vi "QDM matlab saver_morefreqs_rt_2.vi"(6 "img data stack Input":dbl[][](array[numeric]), 7 "matlab path":path, 8 "Height":i64(slide)=1200 min=0 max=1200 step=4 scale=0.0..1200.0, 9 "Width":i64(slide)=1920 min=0 max=1920 step=4 scale=0.0..1920.0, 10 "freq list (Hz)":dbl[](array[numeric]), 11 "sweep #":i32) -> ()   [LabVIEW 2018]
panel:
  in  "numFreqs":i32=51
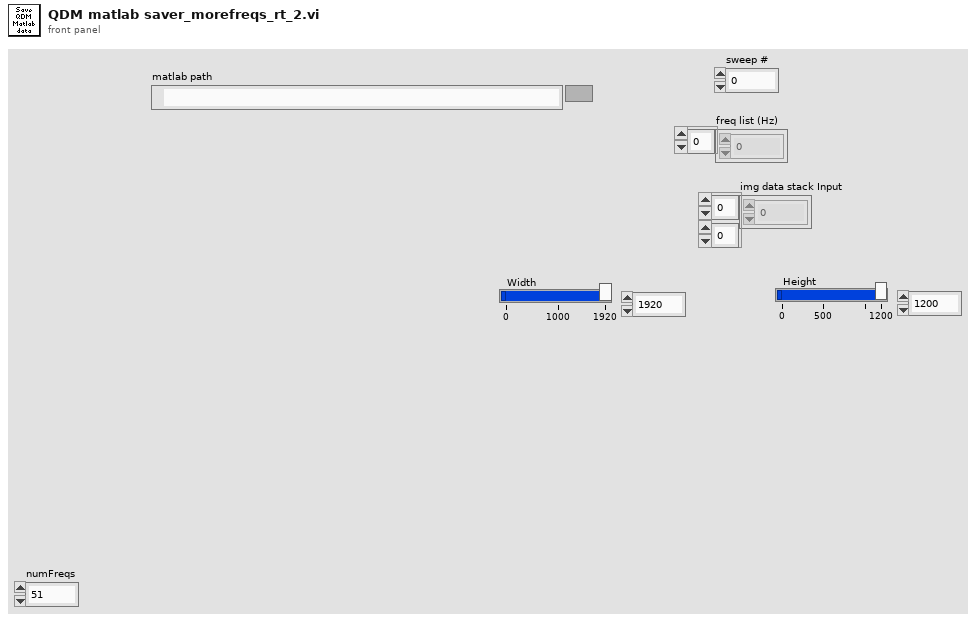
[diagram p1: front panel]
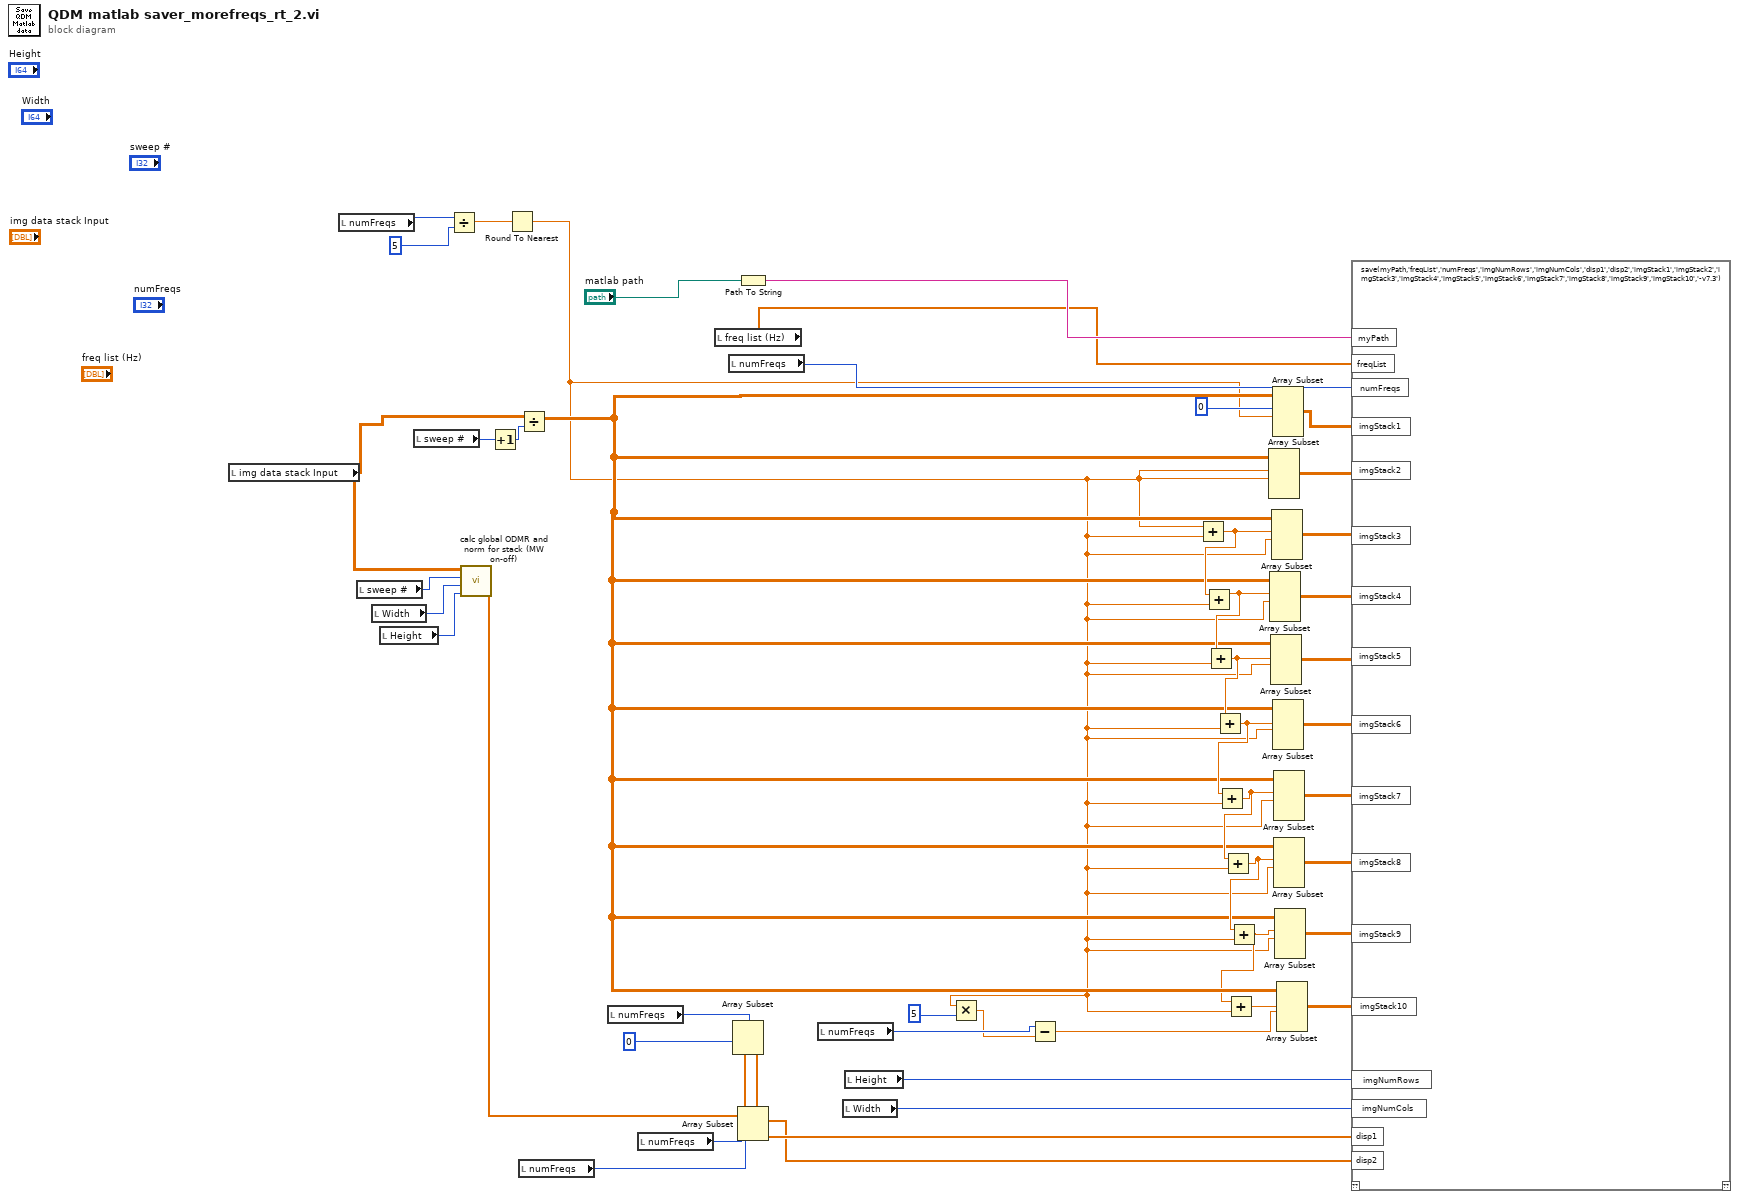
[diagram p0: block diagram]
diagram:
  n1 = local read "img data stack Input"() -> (w37:dbl[][])
  n2 = local read "numFreqs"() -> (w27:i32)
  n3 = local read "sweep #"() -> (w38:i32)
  n4 = local read "Width"() -> (w42:i64)
  n5 = local read "Height"() -> (w43:i64)
  n6 = local read "sweep #"() -> (w40:i32)
  n7 = Divide(x=w27, y=5) -> (x/y=w26:dbl)
  n8 = call "calc global ODMR and norm for stack (MW on-off).vi"("Height"=w43, "Width"=w42, "sweep #"=w38, "img data stack"=w37) -> ("normed spectrum"=w41:dbl[])  [unwired: 7 in]
  n9 = Increment(x=w40) -> (x+1=w39:i32)
  n10 = Round To Nearest(number=w26) -> (nearest integer value=w4:dbl)
  n11 = Divide(x=w37, y=w39) -> (x/y=w12:dbl[][])
  n12 = local read "numFreqs"() -> (w45:i32)
  n13 = local read "numFreqs"() -> (w46:i32)
  n14 = local read "numFreqs"() -> (w44:i32)
  n15 = local read "freq list (Hz)"() -> (w34:dbl[])
  n16 = local read "numFreqs"() -> (w29:i32)
  n17 = Array Subset(array=w41, index=0, length=w46) -> (w31:dbl[])
  n18 = Path To String(path="matlab path") -> (string=w35:string)
  n19 = Array Subset(array=w41, index=w45, length=w44) -> (w30:dbl[])
  n20 = local read "numFreqs"() -> (w3:i32)
  n21 = local read "Width"() -> (w32:i64)
  n22 = local read "Height"() -> (w33:i64)
  n23 = Multiply(x=w4, y=5) -> (x*y=w2:dbl)
  n24 = Subtract(x=w3, y=w2) -> (x-y=w1:dbl)
  n25 = Add(x=w4, y=w4) -> (x+y=w21:dbl)
  n26 = Add(x=w21, y=w4) -> (x+y=w19:dbl)
  n27 = Add(x=w19, y=w4) -> (x+y=w17:dbl)
  n28 = Add(x=w17, y=w4) -> (x+y=w15:dbl)
  n29 = Add(x=w15, y=w4) -> (x+y=w14:dbl)
  n30 = Add(x=w14, y=w4) -> (x+y=w13:dbl)
  n31 = Add(x=w13, y=w4) -> (x+y=w10:dbl)
  n32 = Add(x=w10, y=w4) -> (x+y=w11:dbl)
  n33 = Array Subset(array=w12, index (row)=w4, length (row)=w4) -> (w23:dbl[][])  [unwired: 2 in]
  n34 = Array Subset(array=w12, index (row)=w19, length (row)=w4) -> (w20:dbl[][])  [unwired: 2 in]
  n35 = Array Subset(array=w12, index (row)=w17, length (row)=w4) -> (w18:dbl[][])  [unwired: 2 in]
  n36 = Array Subset(array=w12, index (row)=w21, length (row)=w4) -> (w22:dbl[][])  [unwired: 2 in]
  n37 = Array Subset(array=w12, index (row)=0 ("index"), length (row)=w4) -> (w24:dbl[][])  [unwired: 2 in]
  n38 = Array Subset(array=w12, index (row)=w15, length (row)=w4) -> (w16:dbl[][])  [unwired: 2 in]
  n39 = Array Subset(array=w12, index (row)=w14, length (row)=w4) -> (w9:dbl[][])  [unwired: 2 in]
  n40 = Array Subset(array=w12, index (row)=w13, length (row)=w4) -> (w8:dbl[][])  [unwired: 2 in]
  n41 = Array Subset(array=w12, index (row)=w10, length (row)=w4) -> (w7:dbl[][])  [unwired: 2 in]
  n42 = Array Subset(array=w12, index (row)=w11, length (row)=w1) -> (w6:dbl[][])  [unwired: 2 in]
  n43 = script code="save(myPath,'freqList','numFreqs','imgNumRows','imgNumCols','disp1','disp2','imgStack1','imgStack2','imgStack3','imgStack4','imgStack5','imgStack6','imgStack7','imgStack8','imgStack9','imgStack10','-v7.3')"("myPath"=w35, "freqList"=w34, "imgNumRows"=w33, "imgNumCols"=w32, "disp1"=w31, "disp2"=w30, "numFreqs"=w29, "imgStack1"=w24, "imgStack2"=w23, "imgStack3"=w22, "imgStack4"=w20, "imgStack5"=w18, "imgStack6"=w16, "imgStack7"=w9, "imgStack8"=w8, "imgStack9"=w7, "imgStack10"=w6) -> ()  [unwired: 1 in, 1 out]
